vi "Initialize Devices.vi"(8 "error in (no error)":errorcluster, 11 "Starter Kit host FPGA 2.0 in":refnum<class "NI_Robotics_Starter Kit Host_FPGA_2.0.lvclass">) -> (0 "error out":errorcluster, 3 "Starter Kit host FPGA 2.0 out":refnum<class "NI_Robotics_Starter Kit Host_FPGA_2.0.lvclass">)   [LabVIEW 2017, in "NI_Robotics_Starter Kit Host_FPGA_2.0.lvclass"]
uses:
  <vilib>/robotics/Starter Kit/2.0/FPGA Host Interface/NI_Robotics_Starter Kit Host_FPGA_2.0.lvclass
  c:/Program Files (x86)/National Instruments/LabVIEW 2017/vi.lib/robotics/Starter Kit/Host Interface/NI_Robotics_Starter Kit Host.lvclass
  <vilib>/robotics/Starter Kit/2.0/FPGA Host Interface/NI_Robotics_Starter Kit Host_FPGA_2.0.lvclass/NI_Robotics_Starter Kit Host_FPGA_2.0.ctl
  <vilib>/robotics/Starter Kit/Host Interface/NI_Robotics_Starter Kit Host.lvclass/NI_Robotics_Starter Kit Host.ctl
  <vilib>/robotics/Starter Kit/FPGA Direct IO/NI_Robotics_Starter Kit Direct IO_FPGA.lvclass/NI_Robotics_Starter Kit Direct IO_FPGA.ctl
  <vilib>/robotics/Starter Kit/Base Device/NI_Robotics_Starter Kit Base Device.lvclass/NI_Robotics_Starter Kit Base Device.ctl
  <vilib>/robotics/Starter Kit/Servo Motor 2.0/NI_Robotics_Starter Kit Servo Motor_2.0.lvclass
  c:/Program Files (x86)/National Instruments/LabVIEW 2017/vi.lib/robotics/Starter Kit/Servo Motor/NI_Robotics_Starter Kit Servo Motor.lvclass
  <vilib>/robotics/Starter Kit/FPGA Direct IO/NI_Robotics_Starter Kit Direct IO_FPGA.lvclass
  c:/Program Files (x86)/National Instruments/LabVIEW 2017/vi.lib/robotics/Starter Kit/Base Device/NI_Robotics_Starter Kit Base Device.lvclass
  c:/Program Files (x86)/National Instruments/LabVIEW 2017/vi.lib/robotics/Starter Kit/Direct IO/NI_Robotics_Starter Kit Direct IO.lvclass
  <vilib>/robotics/Starter Kit/Host Interface/NI_Robotics_Starter Kit Host.lvclass
  <instrlib>/DC Motor Controller/HAIOL/FPGA/DC Motor Controller FPGA.lvclass
  <instrlib>/Parallax PING)))/HAIOL/FPGA/Parallax PING))) FPGA.lvclass
  <instrlib>/Hitec HS400 Series/HAIOL/FPGA/Hitec HS400 Series FPGA.lvclass
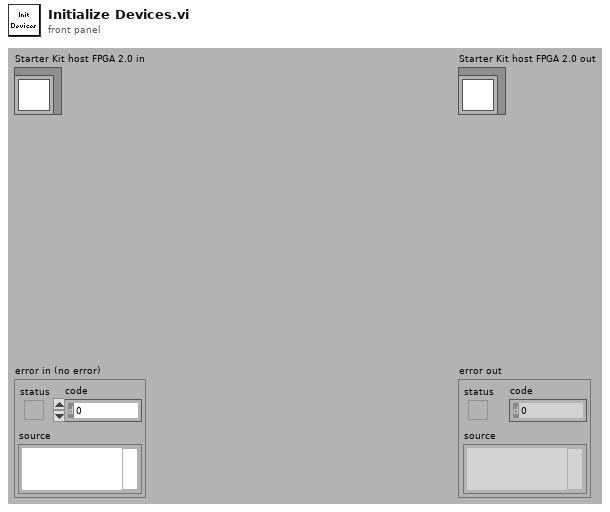
[diagram p1: front panel]
types:
  T1 = typedef "NI_Robotics_Starter Kit Host_FPGA_2.0.lvclass/FPGA Refnum.ctl" = refnum<k20>
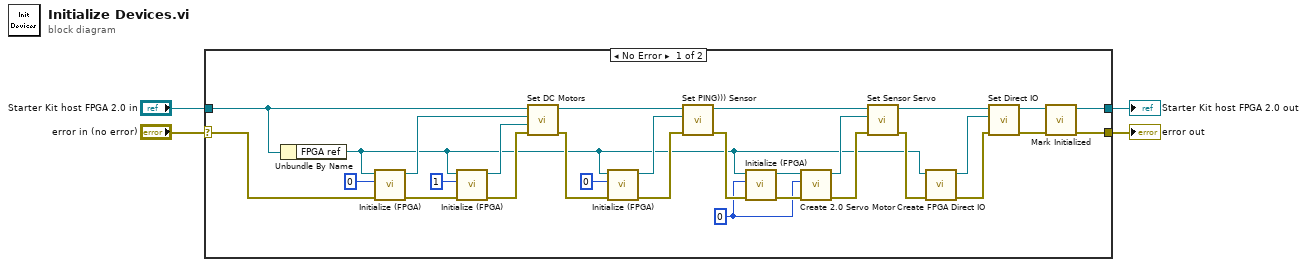
[diagram p0: block diagram]
diagram:
  n1 = case shown="No Error" "error in (no error)" {
    selector: "error in (no error)" -> [w6 w35]
    tunnel: [w5 w35] -> w3
    tunnel: [w10 w34] -> w1
    tunnel: "Starter Kit host FPGA 2.0 in" -> [w9 w34]
    frame No Error {
      w7 = 0 ("servo ID")
      n2 = Unbundle By Name(w9) -> ("FPGA ref"=w8:T1)
      n3 = call <instrlib>:"Initialize (FPGA).vi"("error in (no error)"=w6, "Actuator ID (0)"=u16 0 ("motor ID"), "FPGA VI Reference"=w8) -> ("error out"=w24:errorcluster, "DC Motor Controller out"=w28:refnum<class "DC Motor Controller.lvclass">)  [unwired: 7 in]
      n4 = call <instrlib>:"Initialize (FPGA).vi"("error in (no error)"=w24, "Actuator ID (0)"=u16 1 ("motor ID"), "FPGA VI Reference"=w8) -> ("error out"=w21:errorcluster, "DC Motor Controller out"=w22:refnum<class "DC Motor Controller.lvclass">)  [unwired: 7 in]
      n5 = call <vilib>:"Set DC Motors.vi"("error in (no error)"=w21, "DC motor 1 (right)"=w22, "DC motor 0 (left)"=w28, "NI_Robotics_Starter Kit Host in"=w9) -> ("error out"=w19:errorcluster, "NI_Robotics_Starter Kit Host out"=w18:refnum<class "NI_Robotics_Starter Kit Host_FPGA_2.0.lvclass">)  [unwired: 6 in]
      n6 = call <instrlib>:"Initialize (FPGA).vi"("error in (no error)"=w19, "Sensor ID (0)"=0 ("PING))) ID"), "FPGA VI Reference"=w8) -> ("error out"=w16:errorcluster, "Parallax PING))) out"=w17:refnum<class "Parallax PING))).lvclass">)  [unwired: 7 in]
      n7 = call <vilib>:"Set PING))) Sensor.vi"("error in (no error)"=w16, "PING)))"=w17, "NI_Robotics_Starter Kit Host in"=w18) -> ("error out"=w33:errorcluster, "NI_Robotics_Starter Kit Host out"=w15:refnum<class "NI_Robotics_Starter Kit Host_FPGA_2.0.lvclass">)  [unwired: 7 in]
      n8 = call <instrlib>:"Initialize (FPGA).vi"("error in (no error)"=w33, "Actuator ID (0)"=w7, "FPGA VI Reference"=w8) -> ("error out"=w30:errorcluster, "Hitec HS400 Series out"=w29:refnum<class "Hitec HS400 Series.lvclass">)  [unwired: 7 in]
      n9 = call <vilib>:"Create 2.0 Servo Motor.vi"("error in (no error)"=w30, "servo ID"=w7, "Hitec HS400 servo"=w29) -> ("error out"=w32:errorcluster, "Starter Kit Servo Motor_2.0 out"=w31:refnum<class "NI_Robotics_Starter Kit Servo Motor_2.0.lvclass">)  [unwired: 7 in]
      n10 = call <vilib>:"Set Sensor Servo.vi"("error in (no error)"=w32, "sensor servo"=w31, "NI_Robotics_Starter Kit Host in"=w15) -> ("error out"=w14:errorcluster, "NI_Robotics_Starter Kit Host out"=w13:refnum<class "NI_Robotics_Starter Kit Host_FPGA_2.0.lvclass">)  [unwired: 7 in]
      n11 = call <vilib>:"Create FPGA Direct IO.vi"("error in (no error)"=w14, "FPGA Interface"=w8) -> ("error out"=w11:errorcluster, "FPGA direct IO out"=w12:refnum<class "NI_Robotics_Starter Kit Direct IO_FPGA.lvclass">)  [unwired: 8 in]
      n12 = call <vilib>:"Set Direct IO.vi"("error in (no error)"=w11, "direct IO"=w12, "NI_Robotics_Starter Kit Host in"=w13) -> ("error out"=w26:errorcluster, "NI_Robotics_Starter Kit Host out"=w25:refnum<class "NI_Robotics_Starter Kit Host_FPGA_2.0.lvclass">)  [unwired: 7 in]
      n13 = call <vilib>:"Mark Initialized.vi"("error in (no error)"=w26, "starter kit host in"=w25) -> ("error out"=w5:errorcluster, "starter kit host out"=w10:refnum<class "NI_Robotics_Starter Kit Host_FPGA_2.0.lvclass">)  [unwired: 8 in]
    }
    frame Error {
    }
  }
  "error out" <- w3
  "Starter Kit host FPGA 2.0 out" <- w1
